vi "Test of Display Panel.vi"() -> ()   [LabVIEW 2013]
uses:
  Controls/Numeric Indicator.ctl
  Universal Power Meter/Universal Power Meter class/Universal Power Meter.lvclass
  <vilib>/ActorFramework/Message Queue/Message Queue.lvclass/Message Queue.ctl
  <vilib>/ActorFramework/Message Enqueuer/Message Enqueuer.lvclass/Message Enqueuer.ctl
  <vilib>/ActorFramework/Message Enqueuer/Enqueue.vi
  <vilib>/ActorFramework/Message Priority Queue/Priority Enqueue.vi
  <vilib>/ActorFramework/Actor/Actor.lvclass
  <vilib>/ActorFramework/Stop Msg/Stop Msg.lvclass
  <vilib>/ActorFramework/Message Queue/Message Queue.lvclass
panel:
  out "error out 2":errorcluster
  in  "Card #":dbl format="%#_13g"
  in  "Stop Button":bool
  in  "Enum":enum16{"2", "1"}(ring)
  in  "Numeric Control":i32
  out "error out":errorcluster
  in  "Display Input":T1[](array[typedef])
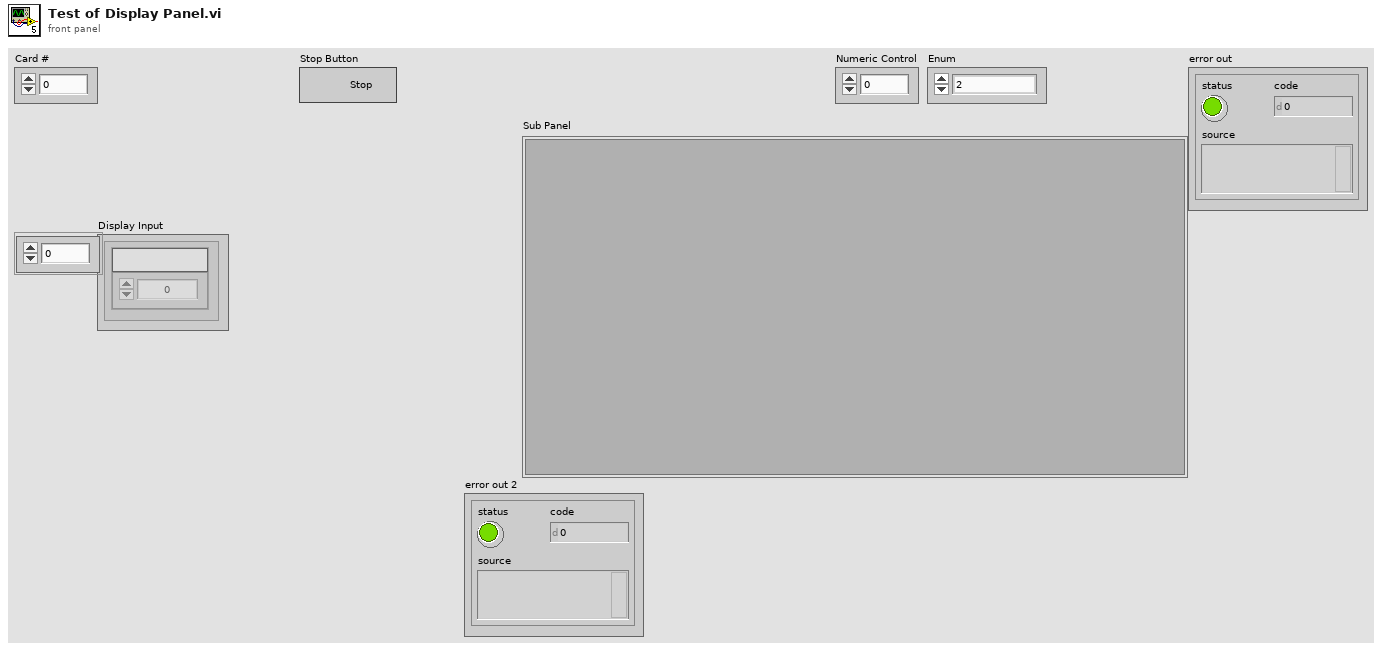
[diagram p1: front panel]
types:
  T1 = typedef "Numeric Indicator.ctl" = cluster{"Numeric Indicator 2":dbl, "String":string}
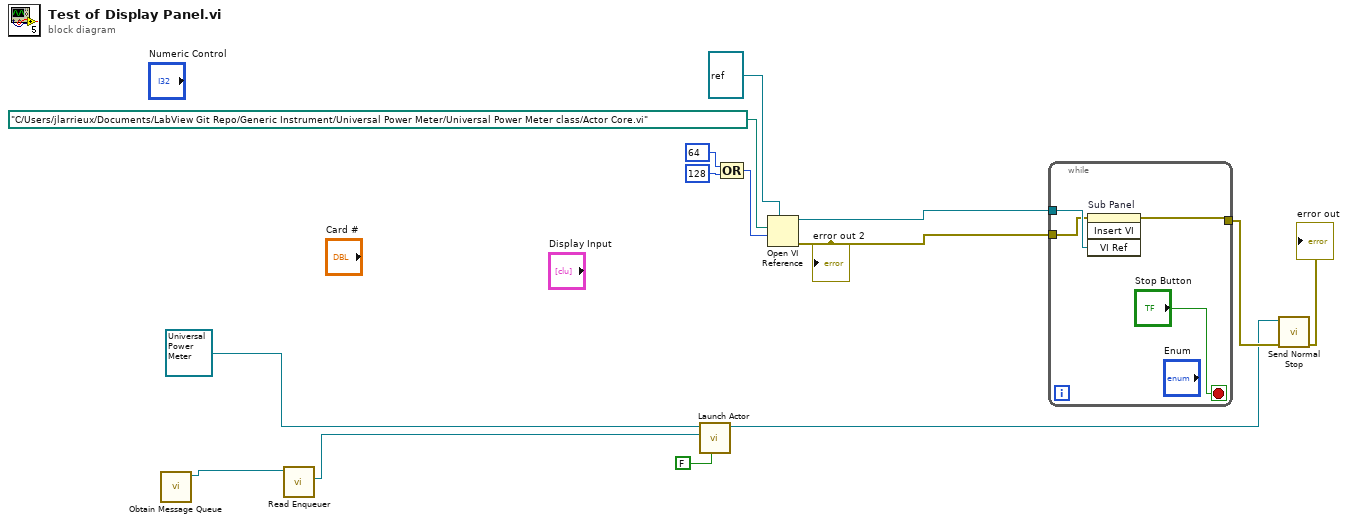
[diagram p0: block diagram]
diagram:
  n1 = call <vilib>:"Obtain Message Queue.vi"() -> ("Message Queue"=w6:refnum<class "Message Queue.lvclass">)  [unwired: 10 in, 1 out]
  n2 = call <vilib>:"Read Enqueuer.vi"("Message Queue"=w6) -> ("Message Enqueuer"=w5:refnum<class "Message Enqueuer.lvclass">)  [unwired: 10 in]
  n3 = call <vilib>:"Launch Actor.vi"("Open Actor Core front panel? (F)"=FALSE, "Actor-to-Caller Enqueuer"=w5, "Actor"=refnum<class "Universal Power Meter.lvclass"> refnum ("Universal Power Meter.lvlib:Universal Power Meter.lvclass")) -> ("Caller-To-Actor Enqueuer"=w3:refnum<class "Message Enqueuer.lvclass">)  [unwired: 7 in, 1 out]
  n4 = Compound Arithmetic op=OR(64 ("options"), 128 ("options")) -> (w10:i32)
  n5 = Open VI Reference(type specifier VI Refnum (for type only)=refnum<vi> refnum, vi path=path "C:/Users/jlarrieux/Documents/LabView Git Repo/Generic Instrument/Universal Power Meter/Universal Power Meter class/Actor Core.vi", options=w10) -> (vi reference=w8:refnum<vi>, error out=w9:errorcluster)  [unwired: 3 in]
  "error out 2" <- w9
  n6 = while {
    tunnel: w8 -> [w17]
    tunnel: w9 -> [w16]
    tunnel: [w15] -> w4
    stop <- "Stop Button" stop-if-true
    n7 = invoke on="Sub Panel" class="SubPanel" method="Insert VI"(error in=w16, "VI Ref"=w17) -> (error out=w15:errorcluster)  [unwired: 2 in, 3 out]
  }
  n8 = call <vilib>:"Send Normal Stop.vi"("error in (no error)"=w4, "Message Enqueuer"=w3) -> ("error out"=→"error out":errorcluster)  [unwired: 9 in]
